vi "calibration equation finder.vi"   [LabVIEW 2019]
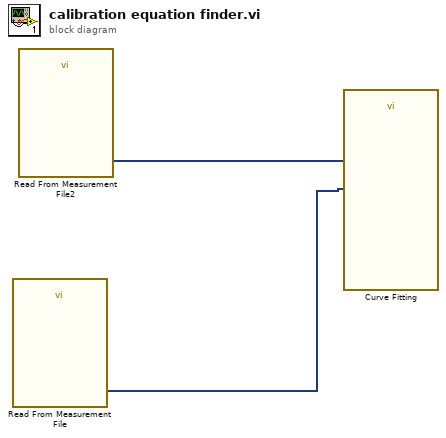
[diagram p0: block diagram]
diagram:
  n1 = call "Read From Measurement File"() -> ("Signals"=w1:dynamicdata)  [unwired: 6 in, 5 out]
  n2 = call "Read From Measurement File2"() -> ("Signals"=w2:dynamicdata)  [unwired: 6 in, 5 out]
  n3 = call "Curve Fitting"("Locations"=w1, "Signals"=w2) -> ()  [unwired: 4 in, 6 out]
